vi "Create CSV.vi"(8 "error in (no error)":errorcluster, 11 "Report in":refnum<class "Report.lvclass">) -> (0 "error out":errorcluster, 2 "CSV":string, 3 "Report out":refnum<class "Report.lvclass">)   [LabVIEW 2024, in "Report.lvclass"]
uses:
  Report.lvclass
  Report.lvclass/Report.ctl
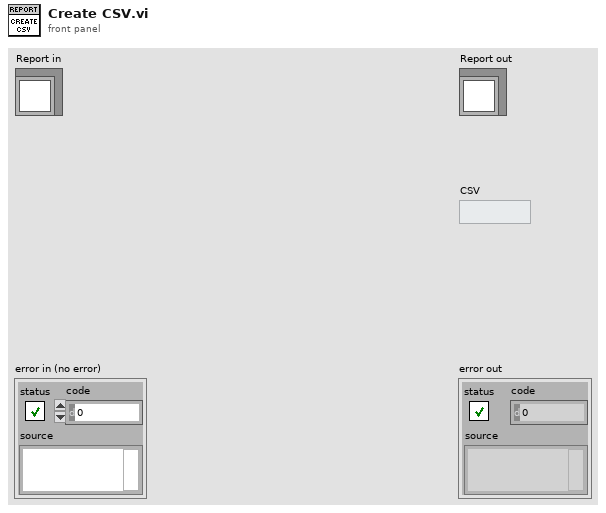
[diagram p1: front panel]
types:
  T1 = typedef "Controller.lvclass/rwr_Get Actual Data Reply.ctl" = cluster{"Temperature [°C]":dbl, "CPU [%]":dbl, "Place":string, "Timestamp":timestamp}
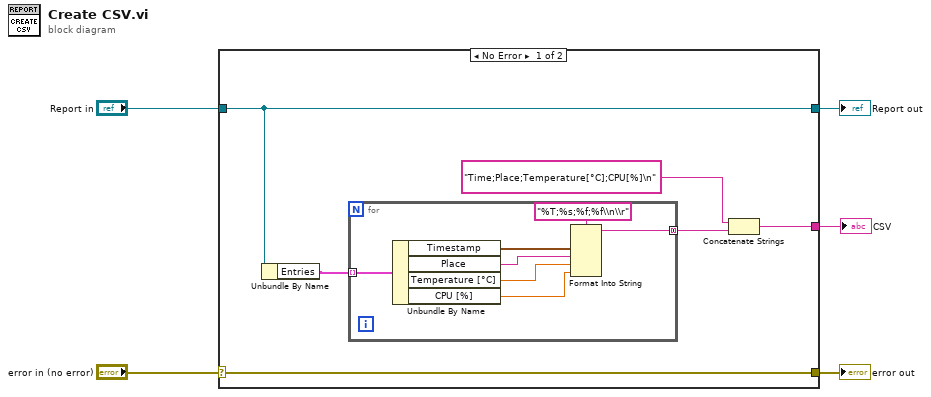
[diagram p0: block diagram]
diagram:
  n1 = case shown="No Error" "error in (no error)" {
    selector: "error in (no error)" -> [w11 w20]
    tunnel: [w11 w20] -> w4
    tunnel: [w10 w19] -> w2
    tunnel: "Report in" -> [w10 w19]
    tunnel: [w7 _] -> w1
    frame No Error {
      n2 = Unbundle By Name(w10) -> ("Entries"=w9:T1[])
      n3 = for {
        tunnel: w9 -> [w18] mode=indexing
        tunnel: [w12] -> w8 mode=concatenating
        n4 = Unbundle By Name(w18) -> ("Timestamp"=w17:timestamp, "Place"=w16:string, "Temperature [°C]"=w15:dbl, "CPU [%]"=w14:dbl)
        n5 = Format Into String(format string="%T;%s;%f;%f\\n\\r", w17, w16, w15, w14) -> (resulting string=w12:string)  [unwired: 2 in, 1 out]
      }
      n6 = Concatenate Strings("Time;Place;Temperature[°C];CPU[%]\n", w8) -> (w7:string)
    }
    frame Error {
    }
  }
  "error out" <- w4
  "Report out" <- w2
  "CSV" <- w1
